vi "simulate_data.vi"() -> (0 "Dados":dbl[](array[numeric]))   [LabVIEW 2016]
uses:
  <vilib>/ptbypt/NI_PtbyPt.lvlib
panel:
  in  "Ruido":dbl(slide) scale=0.0..3e-05 scale format="%#.2p"
  in  "SG 3":dbl(slide) scale=-0.0004..0.0004 scale format="%#.2p"
  in  "SG 2":dbl(slide) scale=-0.0004..0.0004 scale format="%#.2p"
  in  "SG 1":dbl(slide) scale=-0.0004..0.0004 scale format="%#.2p"
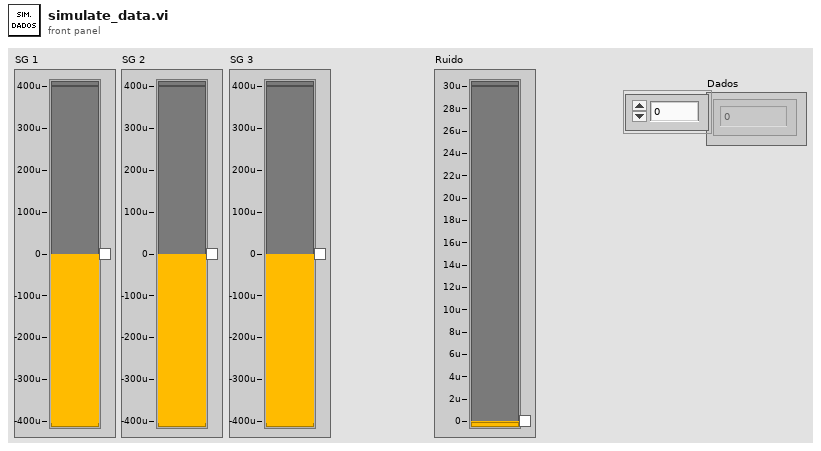
[diagram p1: front panel]
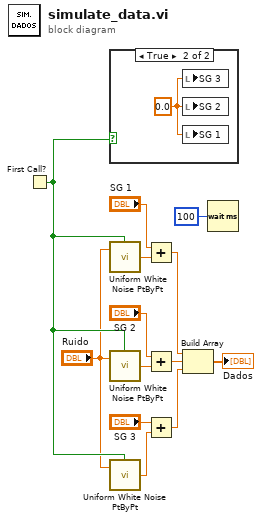
[diagram p0: block diagram]
diagram:
  n1 = First Call?() -> (First Call?: T/F=w12:bool)
  n2 = case shown="True" w12 {
    frame False {
    }
    frame True {
      w14 = 0.0 ("SG 3")
      n3 = local write "SG 3"(w14) -> ()
      n4 = local write "SG 2"(w14) -> ()
      n5 = local write "SG 1"(w14) -> ()
    }
  }
  n6 = call <vilib>:"Uniform White Noise PtByPt.vi"("initialize"=w12, "amplitude"="Ruido") -> ("uniform white noise"=w9:dbl)  [unwired: 1 in]
  n7 = call <vilib>:"Uniform White Noise PtByPt.vi"("initialize"=w12, "amplitude"="Ruido") -> ("uniform white noise"=w7:dbl)  [unwired: 1 in]
  n8 = call <vilib>:"Uniform White Noise PtByPt.vi"("initialize"=w12, "amplitude"="Ruido") -> ("uniform white noise"=w6:dbl)  [unwired: 1 in]
  n9 = Add(x="SG 1", y=w9) -> (x+y=w5:dbl)
  n10 = Add(x="SG 2", y=w7) -> (x+y=w4:dbl)
  n11 = Add(x="SG 3", y=w6) -> (x+y=w3:dbl)
  n12 = Build Array(w5, w4, w3) -> (→"Dados":dbl[])
  n13 = Wait (ms)(milliseconds to wait=u32 100) -> ()  [unwired: 1 out]
